vi "DriveForDistance.vi"() -> ()   [LabVIEW 2019]
uses:
  Framework/Robot Global Data.vi
panel:
  in  "NoWait":bool
  in  "Speed":dbl
  in  "Distance":dbl
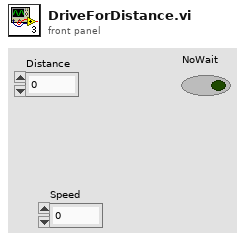
[diagram p1: front panel]
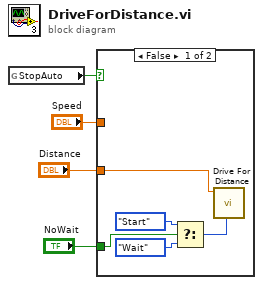
[diagram p0: block diagram]
diagram:
  n1 = global read "Robot Global Data.vi" "StopAuto"() -> (w1:bool)
  n2 = case shown="False" w1 {
    tunnel: "Distance" -> [w5 _]
    tunnel: "Speed" -> [_ _]
    tunnel: "NoWait" -> [w7 _]
    frame False {
      n3 = Select(t=enum16{"Start", "Wait"}."Start" ("Synchronization"), s=w7, f=enum16{"Start", "Wait"}."Wait" ("Synchronization")) -> (s? t:f=w6:enum16{"Start", "Wait"})
      n4 = call "Drive For Distance.vi"("Synchronication"=w6, "Distance"=w5) -> ()  [unwired: 9 in, 1 out]
    }
    frame True {
    }
  }
